vi "Update Switch Button Map.vi"(8 "error in (no error)":errorcluster, 9 "Binding Control Refnums":refnum<vi>[](array[refnum]), 11 "URL Refnum Map In":variant) -> (0 "error out":errorcluster, 3 "URL Refnum Map Out":variant)   [LabVIEW 2024]
doc: "Adds the mapping relationship between the subview switching command and the switch button refnum to the map."
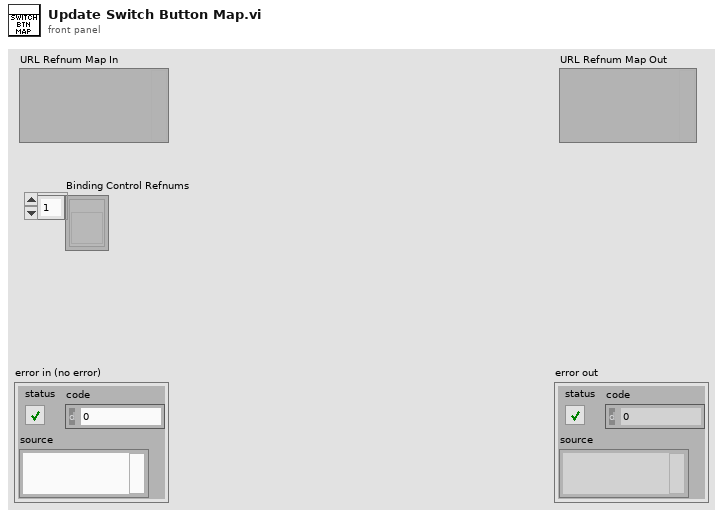
[diagram p1: front panel]
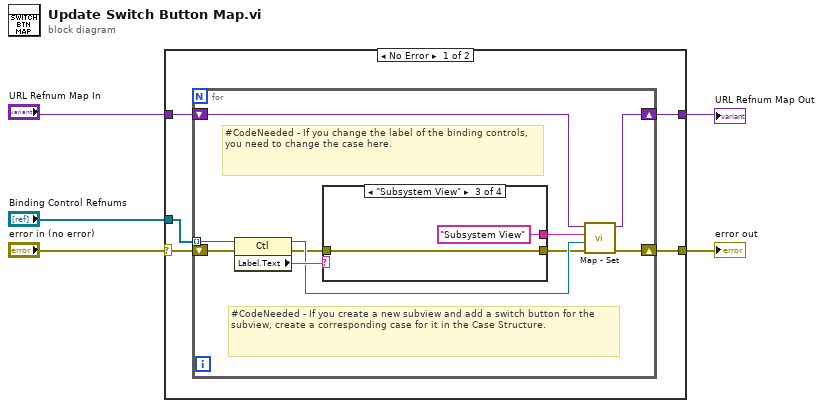
[diagram p0: block diagram]
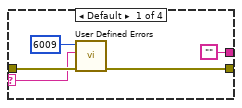
[diagram p2: hidden frame]
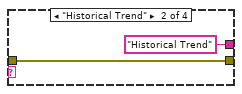
[diagram p3: hidden frame]
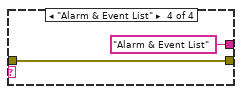
[diagram p4: hidden frame]
diagram:
  n1 = case shown="No Error" "error in (no error)" {
    selector: "error in (no error)" -> [w10 w33]
    tunnel: [w9 w33] -> w4
    tunnel: [w8 w32] -> w3
    tunnel: "URL Refnum Map In" -> [w7 w32]
    tunnel: "Binding Control Refnums" -> [w6 _]
    frame No Error {
      n2 = for {
        tunnel: w6 -> [w20] mode=indexing
        shift-right: [w18] -> w8
        shift-left: w7 -> [w19]
        shift-right: [w17] -> w9
        shift-left: w10 -> [w16]
        # "#CodeNeeded - If you create a new subview and add a switch button for the subview, create a corresponding case for it in the Case Structure."
        # "#CodeNeeded - If you change the label of the binding controls, you need to change the case here."
        n3 = property class="Ctl"(reference=w20, error in=w16) -> (reference out=w14:refnum<vi>, error out=w13:errorcluster, "Label.Text"=w15:string)
        n4 = case shown="\"Subsystem View\"" w15 {
          selector: w15 -> [w22 _ _ _]
          tunnel: ["" "Historical Trend" "Subsystem View" "Alarm & Event List"] -> w12
          tunnel: w13 -> [w24 w27 w29 w31]
          tunnel: [w23 w27 w29 w31] -> w11
          frame Default {
            n5 = call "User Defined Errors.vi"("error in (no error)"=w24, "Parameter 1"=w22, "Error Code (0)"=6009 ("error code (0)")) -> ("error out"=w23:errorcluster)  [unwired: 8 in]
          }
          frame "Historical Trend" {
          }
          frame "Subsystem View" {
          }
          frame "Alarm & Event List" {
          }
        }
        n6 = call "Map - Set.vi"("error in (no error)"=w11, "Value"=w14, "Key"=w12, "Map In"=w19) -> ("error out"=w17:errorcluster, "Map Out"=w18:variant)  [unwired: 5 in, 1 out]
      }
    }
    frame Error {
    }
  }
  "error out" <- w4
  "URL Refnum Map Out" <- w3
